vi "Send.vi"   [LabVIEW 2019, in "DSF Core.lvlib" / "Logging Interface.lvclass"]
uses:
  Logging Interface.lvclass
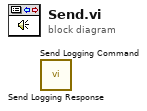
[diagram p0: block diagram]
diagram:
  n1 = call "Send Logging Response.vi"() -> ()  [unwired: 10 in, 2 out]
  n2 = call "Send Logging Command.vi"() -> ()  [unwired: 10 in, 2 out]
